vi "Exp-7.vi"() -> ()   [LabVIEW 2025]
uses:
  <vilib>/express/express arith-compare/Formula/XNode/ExpressFormulaBlockNode.xnode
panel:
  out "Boolean":bool
  out "System rise time in ns":dbl(knob) scale=0.0..10.0
  out "Allowed System rise time delay in ns":dbl(knob) scale=0.0..10.0
  in  "Enum":enum16{"RZ", "NRZ"}(ring)
  in  "Receiver Bandwidth in Ghz":dbl(slide) scale=0.0..10.0
  in  "Rise time Modal (Intermodal) in ns":dbl(slide) scale=0.0..0.1
  in  "Rise time GVD (Intra model) in ns":dbl(slide) scale=0.0..0.1
  in  "Rise time of receiver in ns":dbl(slide) scale=0.0..0.2
  in  "Rise time of transmitter in ns":dbl(slide) scale=0.0..0.1
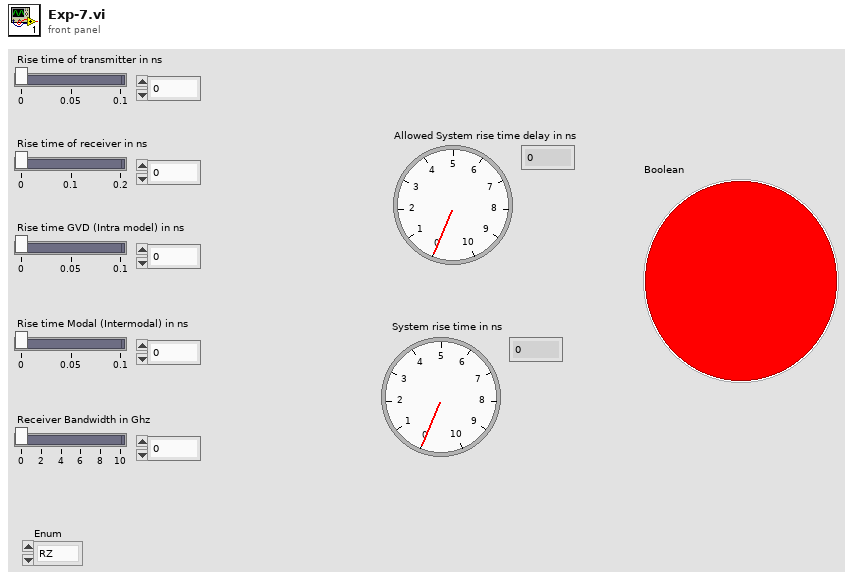
[diagram p1: front panel]
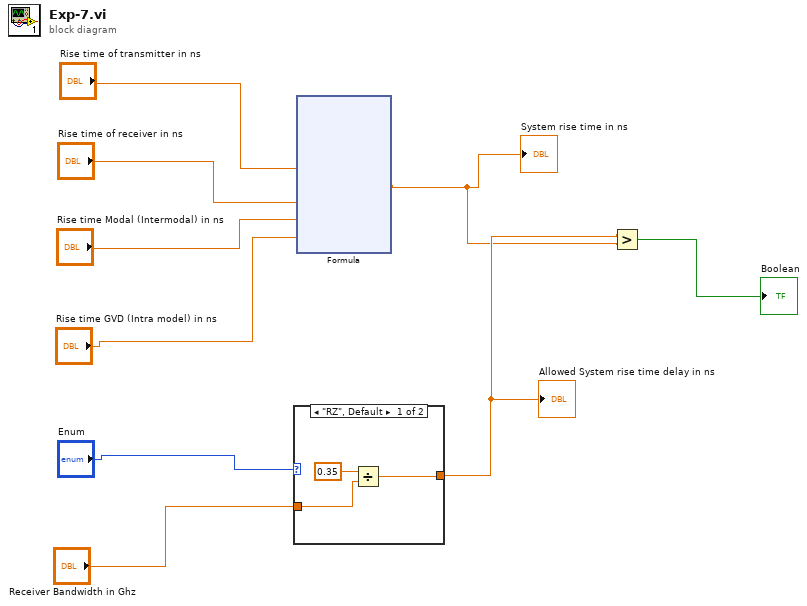
[diagram p0: block diagram]
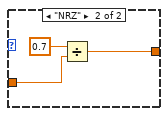
[diagram p2: hidden frame]
diagram:
  n1 = case shown="\"RZ\", Default" "Enum" {
    tunnel: "Receiver Bandwidth in Ghz" -> [w11 w14]
    tunnel: [w10 w13] -> w3
    frame "RZ", Default {
      n2 = Divide(x=0.35, y=w11) -> (x/y=w10:dbl)
    }
    frame "NRZ" {
      n3 = Divide(x=0.7, y=w14) -> (x/y=w13:dbl)
    }
  }
  "Allowed System rise time delay in ns" <- w3
  n4 = xnode "Formula"("Tr"="Rise time of transmitter in ns", "Tt"="Rise time of receiver in ns", "Tmodal"="Rise time Modal (Intermodal) in ns", "Tgvd"="Rise time GVD (Intra model) in ns") -> ("Result"=w2:dbl)  [unwired: 1 in, 1 out]
  "System rise time in ns" <- w2
  n5 = Greater?(x=w3, y=w2) -> (0:→"Boolean":bool)
